vi "PCert-ConfigPageNF-ReadyForSubPanel.vi"(8 "error in (no error)":errorcluster, 11 "ERP-ConfigPageNF in":refnum<class "PCert-ConfigPageNF.lvclass">) -> (0 "error out":errorcluster, 3 "ERP-ConfigPageNF out":refnum<class "PCert-ConfigPageNF.lvclass">)   [LabVIEW 2013, in "PCert-ConfigPageNF.lvclass"]
uses:
  PCert-ConfigPageNF.lvclass
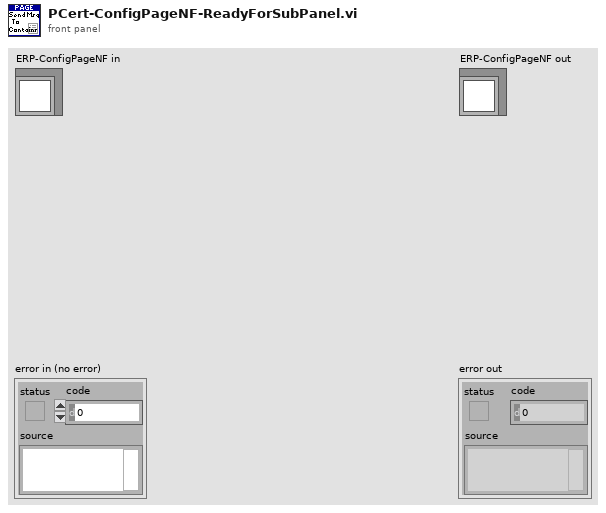
[diagram p1: front panel]
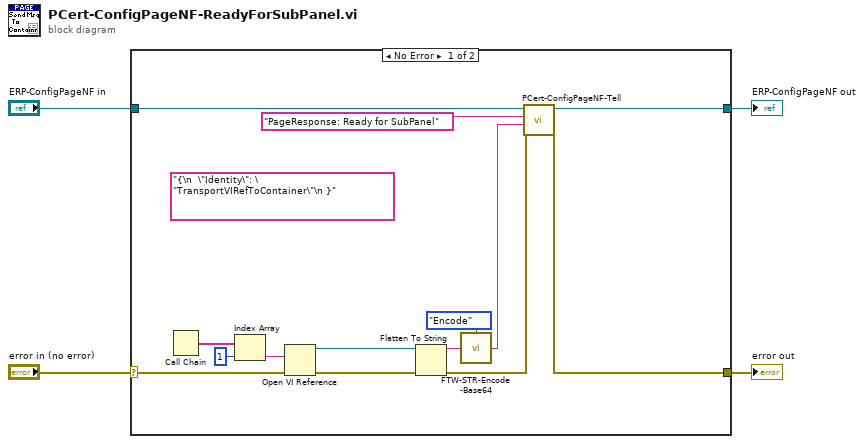
[diagram p0: block diagram]
diagram:
  n1 = case shown="No Error" "error in (no error)" {
    selector: "error in (no error)" -> [w13 w20]
    tunnel: [w12 w20] -> w3
    tunnel: [w14 w19] -> w1
    tunnel: "ERP-ConfigPageNF in" -> [w15 w19]
    frame No Error {
      (unwired) "{\n  \"Identity\": \"TransportVIRefToContainer\"\n }" ("FTW Actor Instance Configuration")
      n2 = Call Chain() -> (call chain=w16:string[])
      n3 = Index Array(array=w16, index=1) -> (element=w18:string)
      n4 = Open VI Reference(vi path=w18, error in (no error)=w13) -> (vi reference=w9:refnum<vi>, error out=w10:errorcluster)  [unwired: 4 in]
      n5 = Flatten To String(anything=w9, error in (no error)=w10) -> (data string=w7:string, error out=w8:errorcluster)  [unwired: 2 in, 1 out]
      n6 = call "FTW-STR-Encode-Base64.vi"("Input"=w7, "Direction"=enum16{"Encode", "Decode"}."Encode") -> ("Output"=w6:string)
      n7 = call "PCert-ConfigPageNF-Tell.vi"("error in (no error)"=w8, "Message Body"=w6, "Message Header"="PageResponse: Ready for SubPanel", "ERP-ConfigPageNF in"=w15) -> ("error out"=w12:errorcluster, "ERP-ConfigPageNF out"=w14:refnum<class "PCert-ConfigPageNF.lvclass">)  [unwired: 6 in]
    }
    frame Error {
    }
  }
  "error out" <- w3
  "ERP-ConfigPageNF out" <- w1
